vi "finishUp.vi"(8 "error in (no error)":errorcluster, 11 "SingleToneRampAction in":refnum<class "SingleToneRampAction.lvclass">) -> (0 "error out":errorcluster, 3 "SingleToneRampAction out":refnum<class "SingleToneRampAction.lvclass">)   [LabVIEW 2009, in "Views.lvlib" / "ScriptEditor.lvlib" / "SingleToneRampAction.lvclass"]
uses:
  SingleToneRampAction.lvclass
  SingleToneRampAction.lvclass/SingleToneRampAction.ctl
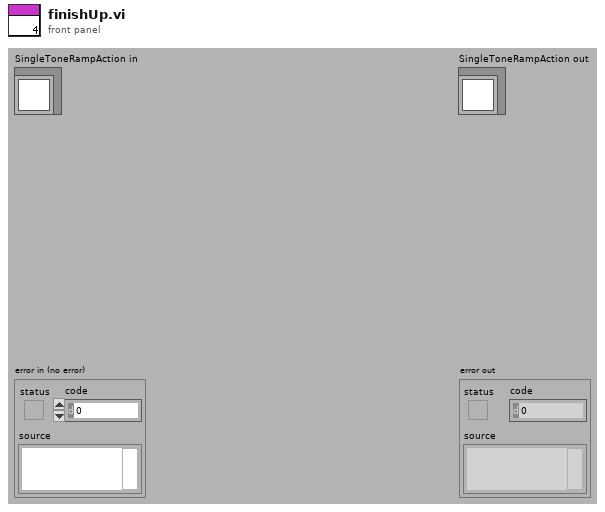
[diagram p1: front panel]
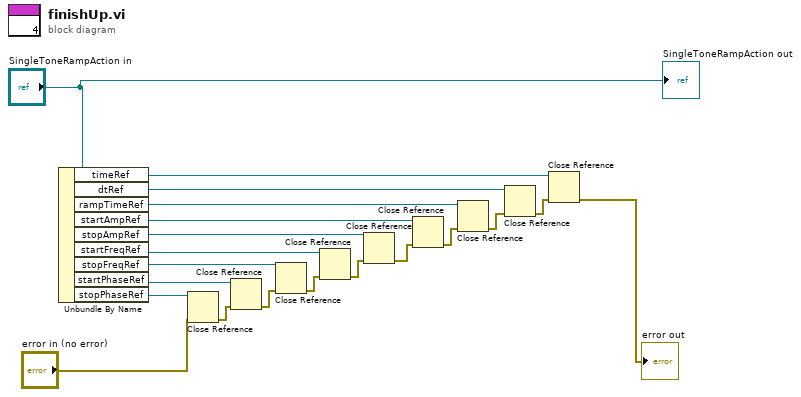
[diagram p0: block diagram]
diagram:
  n1 = Unbundle By Name("SingleToneRampAction in") -> ("timeRef"=w12:refnum<vi>, "dtRef"=w13:refnum<vi>, "rampTimeRef"=w14:refnum<vi>, "startAmpRef"=w15:refnum<vi>, "stopAmpRef"=w16:refnum<vi>, "startFreqRef"=w17:refnum<vi>, "stopFreqRef"=w18:refnum<vi>, "startPhaseRef"=w19:refnum<vi>, "stopPhaseRef"=w20:refnum<vi>)
  n2 = Close Reference(reference=w20, error in (no error)="error in (no error)") -> (error out=w11:errorcluster)
  n3 = Close Reference(reference=w19, error in (no error)=w11) -> (error out=w10:errorcluster)
  n4 = Close Reference(reference=w18, error in (no error)=w10) -> (error out=w9:errorcluster)
  n5 = Close Reference(reference=w17, error in (no error)=w9) -> (error out=w8:errorcluster)
  n6 = Close Reference(reference=w16, error in (no error)=w8) -> (error out=w7:errorcluster)
  n7 = Close Reference(reference=w15, error in (no error)=w7) -> (error out=w6:errorcluster)
  n8 = Close Reference(reference=w14, error in (no error)=w6) -> (error out=w5:errorcluster)
  n9 = Close Reference(reference=w13, error in (no error)=w5) -> (error out=w4:errorcluster)
  n10 = Close Reference(reference=w12, error in (no error)=w4) -> (error out=→"error out":errorcluster)
  "SingleToneRampAction out" <- "SingleToneRampAction in"
